vi "Synth Match Clocks.vi"(9 "F1 Clock mutiplier":u32, 10 "F2":u32, 11 "F1":u32) -> (1 "New clock rate":u32, 2 "New F2":u32, 3 "New F1":u32, 4 "F2 remainder":u32, 5 "F1 remaider":u32)   [LabVIEW 2016]
doc: "This VI should come up with new F1, F2 and Clock integer frequencies, where Clock is divisible by F1 and F2."
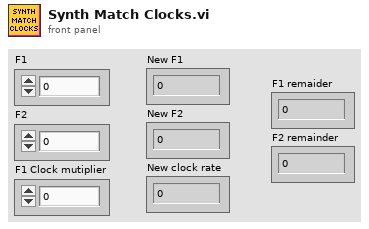
[diagram p1: front panel]
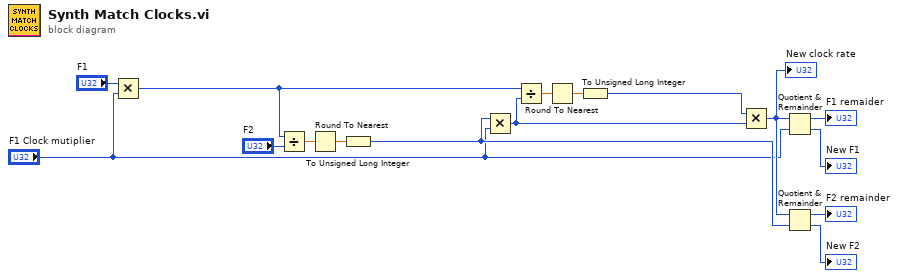
[diagram p0: block diagram]
diagram:
  n1 = Multiply(x="F1", y="F1 Clock mutiplier") -> (x*y=w13:u32)
  n2 = Divide(x=w13, y="F2") -> (x/y=w15:dbl)
  n3 = Round To Nearest(number=w15) -> (nearest integer value=w14:dbl)
  n4 = To Unsigned Long Integer(number=w14) -> (unsigned 32bit integer=w6:u32)
  n5 = Multiply(x=w6, y="F1 Clock mutiplier") -> (x*y=w9:u32)
  n6 = Divide(x=w13, y=w9) -> (x/y=w11:dbl)
  n7 = Round To Nearest(number=w11) -> (nearest integer value=w12:dbl)
  n8 = To Unsigned Long Integer(number=w12) -> (unsigned 32bit integer=w10:u32)
  n9 = Multiply(x=w10, y=w9) -> (x*y=w7:u32)
  "New clock rate" <- w7
  n10 = Quotient & Remainder(x=w7, y="F1 Clock mutiplier") -> (x-y*floor(x/y)=→"F1 remaider":u32, floor(x/y)=→"New F1":u32)
  n11 = Quotient & Remainder(x=w7, y=w6) -> (x-y*floor(x/y)=→"F2 remainder":u32, floor(x/y)=→"New F2":u32)
